vi "Get Data from RAM.vi"(8 "error in (no error)":errorcluster, 9 "End offset":u64, 10 "Start offset":u64, 11 "RP Communicator in":refnum<class "RP Communicator.lvclass">) -> (0 "error out":errorcluster, 2 "data out":string, 3 "RP Communicator out":refnum<class "RP Communicator.lvclass">)   [LabVIEW 2015, in "RP Communicator.lvclass"]
uses:
  RP Communicator.lvclass
  RP Command.ctl
  RP Communicator.lvclass/RP Communicator.ctl
  RP Write Command TCP.vi
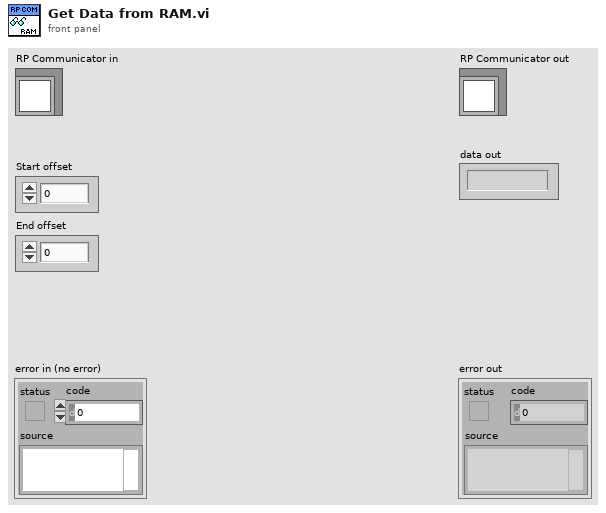
[diagram p1: front panel]
types:
  T1 = typedef "RP Command.ctl" = enum16{"Reset", "Read IDN", "Stop server", "Get status", "Get temperature", "Connect client", "Arm", "Software trigger", "Get whole buffer", "Get chunk", "System call", "Get config", "Set config", "Recieve data", "Play pattern", "Transmit data"}
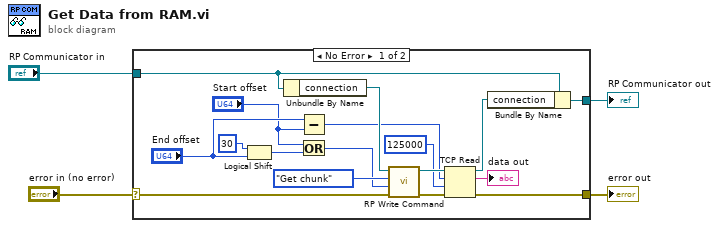
[diagram p0: block diagram]
diagram:
  n1 = case shown="No Error" "error in (no error)" {
    selector: "error in (no error)" -> [w7 w23]
    tunnel: [w6 w23] -> w3
    tunnel: [w9 w22] -> w1
    tunnel: "RP Communicator in" -> [w21 w22]
    frame No Error {
      n2 = Logical Shift(y=i16 30, x="End offset") -> (x << y=w15:u64)
      n3 = Unbundle By Name(w21) -> ("connection"=w20:refnum<k5>)
      n4 = Subtract(x="End offset", y="Start offset") -> (x-y=w11:u64)
      n5 = Or(x="Start offset", y=w15) -> (x .or. y?=w14:u64)
      n6 = call-poly "RP Write Command.vi"("Error In"=w7, "Command payload"=w14, "Command number"=RP_Command."Get chunk", "connection ID"=w20) -> ("Error Out"=w19:errorcluster, "connection ID out"=w18:refnum<k5>)  [unwired: 5 in, 1 out]
      n7 = TCP Read(connection ID=w18, bytes to read=w11, error in (no error)=w19, 9:125000 ("timeout ms (25000)")) -> (connection ID out=w8:refnum<k5>, data out=→"data out":string, error out=w6:errorcluster)  [unwired: 1 in]
      n8 = Bundle By Name(cluster=w21, "connection"=w8) -> (w9:refnum<class "RP Communicator.lvclass">)
    }
    frame Error {
    }
  }
  "error out" <- w3
  "RP Communicator out" <- w1
